vi "car.vi"() -> ()   [LabVIEW 2022 SP3]
uses:
  Control 1.ctl
  Control 2.ctl
  chicken.ctl
  plus_one.ctl
  game_over.ctl
  Control 4.ctl
  tree_control.ctl
panel:
  out "Boolean 12":T1
  in  "chicken":T2
  in  "tree 2":T3
  in  "tree":T3
  in  "tree 5":T3
  in  "tree 4":T3
  out "TOP":i16
  out "SCORE":i16
  in  "stop":bool
  in  "tree 3":T3
  out "Boolean 11":T4
  out "grass 5":T5
  out "grass 4":T5
  out "grass 3":T5
  out "grass 2":T5
  out "grass 1":T5
  out "easy?":bool
  in  "HARD":bool
  in  "EASY":bool
  out "Boolean 10":T6
  in  "v 10":dbl
  in  "v 9":dbl
  out "Boolean 9":T7
  in  "v 8":dbl
  out "Boolean 8":T6
  in  "v 7":dbl
  out "Boolean 7":T7
  out "Boolean 6":T6
  in  "v 6":dbl
  in  "v 5":dbl
  out "Boolean 5":T7
  in  "v 4":dbl
  out "Boolean 4":T6
  in  "v 3":dbl
  out "Boolean 3":T7
  in  "v 2":dbl
  in  "v":dbl
  out "Boolean 2":T6
  out "Boolean":T7
  # "SCORE"
  # "TOP"
  # "Press Arrow Key To Control The Chick\nDon't forget to reset the path of music first."
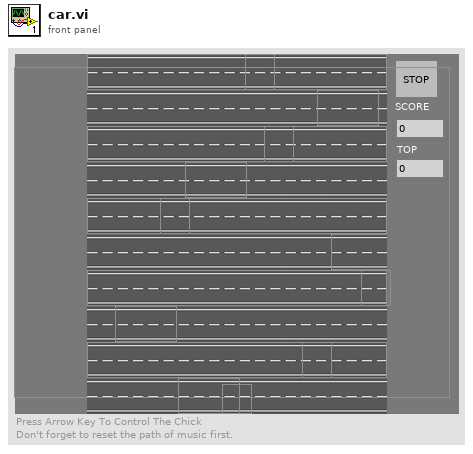
[diagram p1: front panel]
types:
  T1 = typedef "game_over.ctl" = bool
  T2 = typedef "chicken.ctl" = bool
  T3 = typedef "tree_control.ctl" = bool
  T4 = typedef "plus_one.ctl" = bool
  T5 = typedef "Control 4.ctl" = bool
  T6 = typedef "Control 2.ctl" = bool
  T7 = typedef "Control 1.ctl" = bool
  T8 = typedef "Sound Output Task ID.ctl" = u32
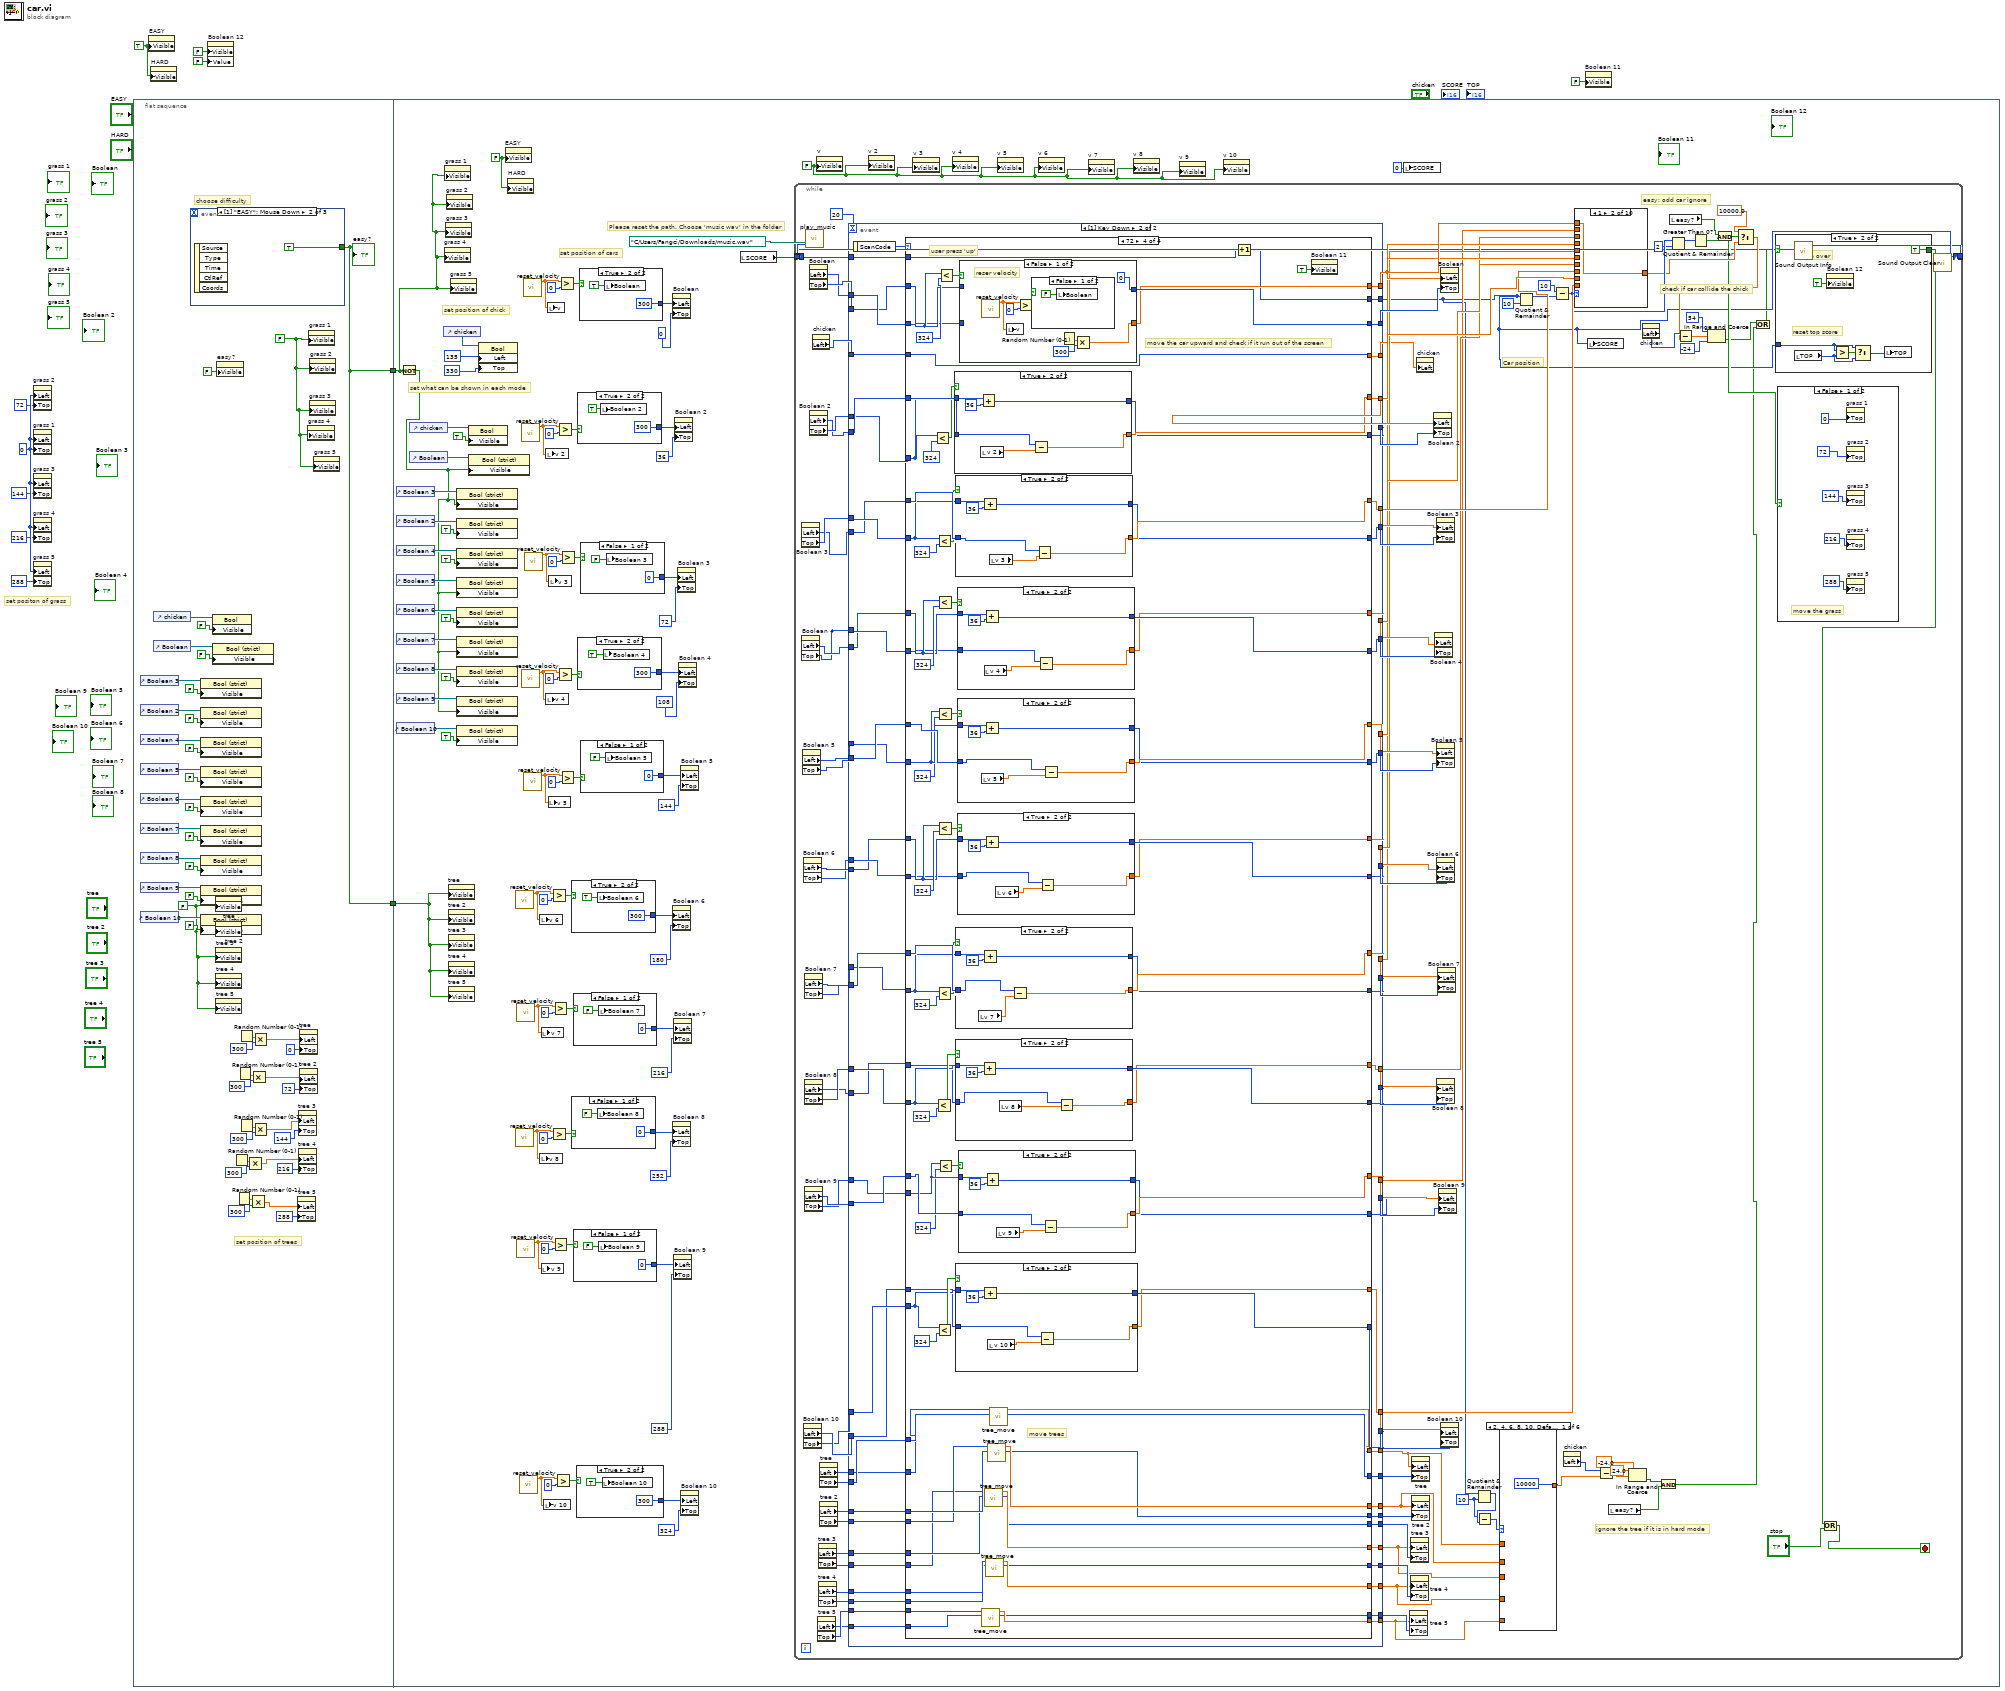
[diagram p0: block diagram]
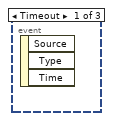
[diagram p2: hidden frame]
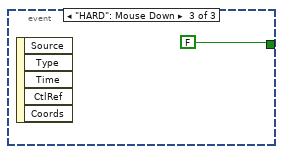
[diagram p3: hidden frame]
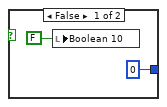
[diagram p4: hidden frame]
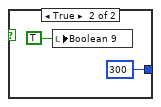
[diagram p5: hidden frame]
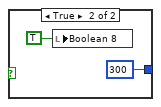
[diagram p6: hidden frame]
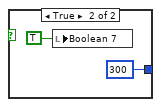
[diagram p7: hidden frame]
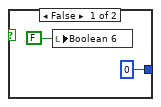
[diagram p8: hidden frame]
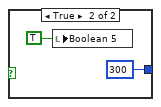
[diagram p9: hidden frame]
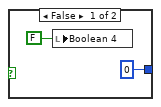
[diagram p10: hidden frame]
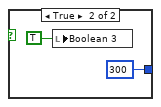
[diagram p11: hidden frame]
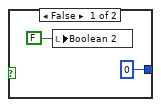
[diagram p12: hidden frame]
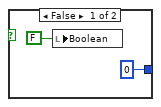
[diagram p13: hidden frame]
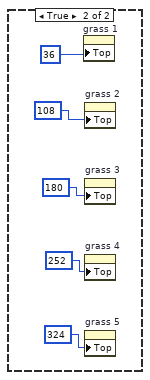
[diagram p19: hidden frame]
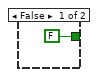
[diagram p20: hidden frame]
diagram:
  w6 = 0
  w8 = TRUE ("Visible")
  # "set positon of grass"
  n1 = property on="grass 2" class="Bool"("Left"=w6, "Top"=72) -> ()  [unwired: 2 in, 2 out]
  n2 = property on="grass 1" class="Bool"("Left"=w6, "Top"=w6) -> ()  [unwired: 2 in, 2 out]
  n3 = property on="grass 3" class="Bool"("Left"=w6, "Top"=144) -> ()  [unwired: 2 in, 2 out]
  n4 = property on="grass 4" class="Bool"("Left"=w6, "Top"=216) -> ()  [unwired: 2 in, 2 out]
  n5 = property on="grass 5" class="Bool"("Left"=w6, "Top"=288) -> ()  [unwired: 2 in, 2 out]
  n6 = flat-sequence {
    tunnel: [w32] -> w7
    tunnel: [w32] -> w1
    tunnel: w7 -> [w65]
    tunnel: w1 -> [w63]
    frame #0 {
      w33 = FALSE
      w34 = FALSE ("Visible")
      # "set position of trees"
      # "choose difficulty"
      n7 = control-ref of="Boolean 3"() -> (w44:refnum<vi>)
      n8 = control-ref of="Boolean 2"() -> (w43:refnum<vi>)
      n9 = control-ref of="Boolean 4"() -> (w42:refnum<vi>)
      n10 = control-ref of="Boolean 5"() -> (w41:refnum<vi>)
      n11 = control-ref of="Boolean 6"() -> (w40:refnum<vi>)
      n12 = control-ref of="Boolean 7"() -> (w39:refnum<vi>)
      n13 = control-ref of="Boolean 8"() -> (w38:refnum<vi>)
      n14 = control-ref of="Boolean 9"() -> (w37:refnum<vi>)
      n15 = control-ref of="Boolean 10"() -> (w35:refnum<vi>)
      n16 = control-ref of="chicken"() -> (w56:refnum<vi>)
      n17 = control-ref of="Boolean"() -> (w45:refnum<vi>)
      n18 = event shown="[1] \"EASY\": Mouse Down" {
        selector: _ -> [_ _ _]
        dyn-events: _ -> [_ _ _]
        timeout: _ -> [_ _ _]
        tunnel: [_ TRUE FALSE] -> w32
        event Timeout {
          n19 = event-data() -> ()  [unwired: 1 in, 3 out]
        }
        event "EASY": Mouse Down {
          n20 = event-data() -> ()  [unwired: 1 in, 5 out]
        }
        event "HARD": Mouse Down {
          n21 = event-data() -> ()  [unwired: 1 in, 5 out]
        }
      }
      "easy?" <- w32
      n22 = property class="Bool (strict)"(reference=w44, "Visible"=FALSE) -> ()  [unwired: 1 in, 2 out]
      n23 = property class="Bool (strict)"(reference=w43, "Visible"=FALSE) -> ()  [unwired: 1 in, 2 out]
      n24 = property class="Bool (strict)"(reference=w42, "Visible"=FALSE) -> ()  [unwired: 1 in, 2 out]
      n25 = property class="Bool (strict)"(reference=w41, "Visible"=FALSE) -> ()  [unwired: 1 in, 2 out]
      n26 = property class="Bool (strict)"(reference=w40, "Visible"=FALSE) -> ()  [unwired: 1 in, 2 out]
      n27 = property class="Bool (strict)"(reference=w39, "Visible"=FALSE) -> ()  [unwired: 1 in, 2 out]
      n28 = property class="Bool (strict)"(reference=w38, "Visible"=FALSE) -> ()  [unwired: 1 in, 2 out]
      n29 = property class="Bool (strict)"(reference=w37, "Visible"=FALSE) -> ()  [unwired: 1 in, 2 out]
      n30 = property class="Bool (strict)"(reference=w35, "Visible"=FALSE) -> ()  [unwired: 1 in, 2 out]
      n31 = property class="Bool"(reference=w56, "Visible"=FALSE) -> ()  [unwired: 1 in, 2 out]
      n32 = property class="Bool (strict)"(reference=w45, "Visible"=FALSE) -> ()  [unwired: 1 in, 2 out]
      n33 = property on="tree" class="Bool"("Visible"=w33) -> ()  [unwired: 2 in, 2 out]
      n34 = property on="tree 2" class="Bool"("Visible"=w33) -> ()  [unwired: 2 in, 2 out]
      n35 = property on="tree 3" class="Bool"("Visible"=w33) -> ()  [unwired: 2 in, 2 out]
      n36 = property on="tree 4" class="Bool"("Visible"=w33) -> ()  [unwired: 2 in, 2 out]
      n37 = property on="tree 5" class="Bool"("Visible"=w33) -> ()  [unwired: 2 in, 2 out]
      n38 = property on="easy?" class="Bool (strict)"("Visible"=FALSE) -> ()  [unwired: 2 in, 2 out]
      n39 = Random Number (0-1)() -> (number: 0 to 1=w23:dbl)
      n40 = Random Number (0-1)() -> (number: 0 to 1=w22:dbl)
      n41 = Random Number (0-1)() -> (number: 0 to 1=w27:dbl)
      n42 = Random Number (0-1)() -> (number: 0 to 1=w31:dbl)
      n43 = Random Number (0-1)() -> (number: 0 to 1=w26:dbl)
      n44 = Multiply(x=w23, y=300) -> (x*y=w18:dbl)
      n45 = Multiply(x=w22, y=300) -> (x*y=w17:dbl)
      n46 = Multiply(x=w27, y=300) -> (x*y=w20:dbl)
      n47 = Multiply(x=w31, y=300) -> (x*y=w29:dbl)
      n48 = Multiply(x=w26, y=300) -> (x*y=w19:dbl)
      n49 = property on="tree 5" class="Bool"("Left"=w17, "Top"=288 ("Position:Top")) -> ()  [unwired: 2 in, 2 out]
      n50 = property on="tree 3" class="Bool"("Left"=w19, "Top"=144 ("Position:Top")) -> ()  [unwired: 2 in, 2 out]
      n51 = property on="tree 4" class="Bool"("Left"=w18, "Top"=216 ("Position:Top")) -> ()  [unwired: 2 in, 2 out]
      n52 = property on="tree" class="Bool"("Left"=w29, "Top"=0 ("Position:Top")) -> ()  [unwired: 2 in, 2 out]
      n53 = property on="tree 2" class="Bool"("Left"=w20, "Top"=72 ("Position:Top")) -> ()  [unwired: 2 in, 2 out]
      n54 = property on="grass 4" class="Bool"("Visible"=w34) -> ()  [unwired: 2 in, 2 out]
      n55 = property on="grass 1" class="Bool"("Visible"=w34) -> ()  [unwired: 2 in, 2 out]
      n56 = property on="grass 3" class="Bool"("Visible"=w34) -> ()  [unwired: 2 in, 2 out]
      n57 = property on="grass 2" class="Bool"("Visible"=w34) -> ()  [unwired: 2 in, 2 out]
      n58 = property on="grass 5" class="Bool"("Visible"=w34) -> ()  [unwired: 2 in, 2 out]
    }
    frame #1 {
      w84 = FALSE ("Visible")
      w98 = FALSE ("Visible")
      # "Please reset the path. Choose 'music wav' in the folder"
      # "set position of cars"
      # "set position of chick"
      # "set what can be shown in each mode"
      n59 = control-ref of="Boolean 3"() -> (w74:refnum<vi>)
      n60 = control-ref of="Boolean 2"() -> (w75:refnum<vi>)
      n61 = control-ref of="Boolean 4"() -> (w76:refnum<vi>)
      n62 = control-ref of="Boolean 5"() -> (w77:refnum<vi>)
      n63 = control-ref of="Boolean 6"() -> (w78:refnum<vi>)
      n64 = control-ref of="Boolean 7"() -> (w79:refnum<vi>)
      n65 = control-ref of="Boolean 8"() -> (w80:refnum<vi>)
      n66 = control-ref of="Boolean 9"() -> (w81:refnum<vi>)
      n67 = control-ref of="Boolean 10"() -> (w83:refnum<vi>)
      n68 = Not(x=w65) -> (.not. x?=w66:bool)
      n69 = control-ref of="chicken"() -> (w67:refnum<vi>)
      n70 = control-ref of="Boolean"() -> (w73:refnum<vi>)
      n71 = control-ref of="chicken"() -> (w88:refnum<vi>)
      n72 = property on="grass 4" class="Bool"("Visible"=w65) -> ()  [unwired: 2 in, 2 out]
      n73 = property on="grass 1" class="Bool"("Visible"=w65) -> ()  [unwired: 2 in, 2 out]
      n74 = property on="grass 3" class="Bool"("Visible"=w65) -> ()  [unwired: 2 in, 2 out]
      n75 = property on="grass 2" class="Bool"("Visible"=w65) -> ()  [unwired: 2 in, 2 out]
      n76 = property on="tree" class="Bool"("Visible"=w63) -> ()  [unwired: 2 in, 2 out]
      n77 = property on="tree 2" class="Bool"("Visible"=w63) -> ()  [unwired: 2 in, 2 out]
      n78 = property on="tree 3" class="Bool"("Visible"=w63) -> ()  [unwired: 2 in, 2 out]
      n79 = property on="tree 4" class="Bool"("Visible"=w63) -> ()  [unwired: 2 in, 2 out]
      n80 = property on="tree 5" class="Bool"("Visible"=w63) -> ()  [unwired: 2 in, 2 out]
      n81 = property on="grass 5" class="Bool"("Visible"=w65) -> ()  [unwired: 2 in, 2 out]
      n82 = property class="Bool (strict)"(reference=w74, "Visible"=w66) -> ()  [unwired: 1 in, 2 out]
      n83 = property class="Bool (strict)"(reference=w75, "Visible"=TRUE) -> ()  [unwired: 1 in, 2 out]
      n84 = property class="Bool (strict)"(reference=w76, "Visible"=TRUE) -> ()  [unwired: 1 in, 2 out]
      n85 = property class="Bool (strict)"(reference=w77, "Visible"=w66) -> ()  [unwired: 1 in, 2 out]
      n86 = property class="Bool (strict)"(reference=w78, "Visible"=TRUE) -> ()  [unwired: 1 in, 2 out]
      n87 = property class="Bool (strict)"(reference=w79, "Visible"=w66) -> ()  [unwired: 1 in, 2 out]
      n88 = property class="Bool (strict)"(reference=w80, "Visible"=TRUE) -> ()  [unwired: 1 in, 2 out]
      n89 = property class="Bool (strict)"(reference=w81, "Visible"=w66) -> ()  [unwired: 1 in, 2 out]
      n90 = property class="Bool (strict)"(reference=w83, "Visible"=TRUE) -> ()  [unwired: 1 in, 2 out]
      n91 = property class="Bool"(reference=w67, "Visible"=TRUE) -> ()  [unwired: 1 in, 2 out]
      n92 = property class="Bool (strict)"(reference=w73, "Visible"=w66) -> ()  [unwired: 1 in, 2 out]
      n93 = property on="Property Node" class="Bool"(reference=w88, "Left"=135 ("Position:Left"), "Top"=330 ("Position:Top")) -> ()  [unwired: 1 in, 2 out]
      n94 = property on="EASY" class="Bool"("Visible"=w84) -> ()  [unwired: 2 in, 2 out]
      n95 = property on="HARD" class="Bool"("Visible"=w84) -> ()  [unwired: 2 in, 2 out]
      n96 = call "reset_velocity.vi"() -> ("Numeric"=w93:dbl)  [unwired: 11 in]
      n97 = call "reset_velocity.vi"() -> ("Numeric"=w91:dbl)  [unwired: 11 in]
      n98 = call "reset_velocity.vi"() -> ("Numeric"=w92:dbl)  [unwired: 11 in]
      n99 = call "reset_velocity.vi"() -> ("Numeric"=w90:dbl)  [unwired: 11 in]
      n100 = call "reset_velocity.vi"() -> ("Numeric"=w89:dbl)  [unwired: 11 in]
      n101 = call "reset_velocity.vi"() -> ("Numeric"=w97:dbl)  [unwired: 11 in]
      n102 = call "reset_velocity.vi"() -> ("Numeric"=w95:dbl)  [unwired: 11 in]
      n103 = call "reset_velocity.vi"() -> ("Numeric"=w139:dbl)  [unwired: 11 in]
      n104 = call "reset_velocity.vi"() -> ("Numeric"=w94:dbl)  [unwired: 11 in]
      n105 = call "reset_velocity.vi"() -> ("Numeric"=w96:dbl)  [unwired: 11 in]
      n106 = local write "v 6"(w93) -> ()
      n107 = local write "v 8"(w91) -> ()
      n108 = local write "v 7"(w92) -> ()
      n109 = local write "v 9"(w90) -> ()
      n110 = local write "v 10"(w89) -> ()
      n111 = local write "v 2"(w97) -> ()
      n112 = local write "v 4"(w95) -> ()
      n113 = local write "v"(w139) -> ()
      n114 = local write "v 5"(w94) -> ()
      n115 = local write "v 3"(w96) -> ()
      n116 = Greater?(x=w93, y=0) -> (0:w118:bool)
      n117 = Greater?(x=w91, y=0) -> (0:w110:bool)
      n118 = Greater?(x=w92, y=0) -> (0:w113:bool)
      n119 = Greater?(x=w90, y=0) -> (0:w105:bool)
      n120 = Greater?(x=w89, y=0) -> (0:w102:bool)
      n121 = Greater?(x=w97, y=0) -> (0:w134:bool)
      n122 = Greater?(x=w95, y=0) -> (0:w126:bool)
      n123 = Greater?(x=w139, y=0) -> (0:w137:bool)
      n124 = Greater?(x=w94, y=0) -> (0:w121:bool)
      n125 = Greater?(x=w96, y=0) -> (0:w129:bool)
      n126 = case shown="True" w118 {
        tunnel: [0 300] -> w116
        frame False {
          n127 = local write "Boolean 6"(FALSE) -> ()
        }
        frame True {
          n128 = local write "Boolean 6"(TRUE) -> ()
        }
      }
      n129 = case shown="False" w110 {
        tunnel: [0 300] -> w108
        frame False {
          n130 = local write "Boolean 8"(FALSE) -> ()
        }
        frame True {
          n131 = local write "Boolean 8"(TRUE) -> ()
        }
      }
      n132 = case shown="False" w113 {
        tunnel: [0 300] -> w112
        frame False {
          n133 = local write "Boolean 7"(FALSE) -> ()
        }
        frame True {
          n134 = local write "Boolean 7"(TRUE) -> ()
        }
      }
      n135 = case shown="False" w105 {
        tunnel: [0 300] -> w104
        frame False {
          n136 = local write "Boolean 9"(FALSE) -> ()
        }
        frame True {
          n137 = local write "Boolean 9"(TRUE) -> ()
        }
      }
      n138 = case shown="True" w102 {
        tunnel: [0 300] -> w100
        frame False {
          n139 = local write "Boolean 10"(FALSE) -> ()
        }
        frame True {
          n140 = local write "Boolean 10"(TRUE) -> ()
        }
      }
      n141 = case shown="True" w134 {
        tunnel: [0 300] -> w132
        frame False {
          n142 = local write "Boolean 2"(FALSE) -> ()
        }
        frame True {
          n143 = local write "Boolean 2"(TRUE) -> ()
        }
      }
      n144 = case shown="True" w126 {
        tunnel: [0 300] -> w124
        frame False {
          n145 = local write "Boolean 4"(FALSE) -> ()
        }
        frame True {
          n146 = local write "Boolean 4"(TRUE) -> ()
        }
      }
      n147 = case shown="True" w137 {
        tunnel: [0 300] -> w136
        frame False {
          n148 = local write "Boolean"(FALSE) -> ()
        }
        frame True {
          n149 = local write "Boolean"(TRUE) -> ()
        }
      }
      n150 = case shown="False" w121 {
        tunnel: [0 300] -> w120
        frame False {
          n151 = local write "Boolean 5"(FALSE) -> ()
        }
        frame True {
          n152 = local write "Boolean 5"(TRUE) -> ()
        }
      }
      n153 = case shown="False" w129 {
        tunnel: [0 300] -> w127
        frame False {
          n154 = local write "Boolean 3"(FALSE) -> ()
        }
        frame True {
          n155 = local write "Boolean 3"(TRUE) -> ()
        }
      }
      n156 = property on="Boolean" class="Bool (strict)"("Left"=w136, "Top"=0) -> ()  [unwired: 2 in, 2 out]
      n157 = property on="Boolean 6" class="Bool (strict)"("Left"=w116, "Top"=180) -> ()  [unwired: 2 in, 2 out]
      n158 = property on="Boolean 8" class="Bool (strict)"("Left"=w108, "Top"=252) -> ()  [unwired: 2 in, 2 out]
      n159 = property on="Boolean 7" class="Bool (strict)"("Left"=w112, "Top"=216) -> ()  [unwired: 2 in, 2 out]
      n160 = property on="Boolean 9" class="Bool (strict)"("Left"=w104, "Top"=288) -> ()  [unwired: 2 in, 2 out]
      n161 = property on="Boolean 2" class="Bool (strict)"("Left"=w132, "Top"=36) -> ()  [unwired: 2 in, 2 out]
      n162 = property on="Boolean 3" class="Bool (strict)"("Left"=w127, "Top"=72) -> ()  [unwired: 2 in, 2 out]
      n163 = property on="Boolean 4" class="Bool (strict)"("Left"=w124, "Top"=108) -> ()  [unwired: 2 in, 2 out]
      n164 = property on="Boolean 5" class="Bool (strict)"("Left"=w120, "Top"=144) -> ()  [unwired: 2 in, 2 out]
      n165 = property on="Boolean 10" class="Bool (strict)"("Left"=w100, "Top"=324) -> ()  [unwired: 2 in, 2 out]
      n166 = local read "SCORE"() -> (w64:i16)
      n167 = call "play_music.vi"("Sound File Path"=path "C:/Users/Fangci/Downloads/music.wav") -> ("task ID"=w61:T8)  [unwired: 10 in]
      n168 = while {
        shift-right: [w201] -> _
        shift-left: w64 -> [w217]
        tunnel: w61 -> [w181]
        tunnel: [w180] -> w60
        stop <- w182 stop-if-true
        w199 = i16 10 ("y")
        # "ignore the tree if it is in hard mode"
        # "check if car collide the chick"
        # "easy: odd car ignore"
        # "Car position"
        n169 = property on="Boolean 3" class="Bool (strict)"() -> ("Left"=w270:i32, "Top"=w271:i32)  [unwired: 2 in, 2 out]
        n170 = property on="Boolean 4" class="Bool (strict)"() -> ("Left"=w268:i32, "Top"=w267:i32)  [unwired: 2 in, 2 out]
        n171 = property on="Boolean 5" class="Bool (strict)"() -> ("Left"=w257:i32, "Top"=w265:i32)  [unwired: 2 in, 2 out]
        n172 = property on="Boolean 6" class="Bool (strict)"() -> ("Left"=w263:i32, "Top"=w262:i32)  [unwired: 2 in, 2 out]
        n173 = property on="Boolean 10" class="Bool (strict)"() -> ("Left"=w250:i32, "Top"=w249:i32)  [unwired: 2 in, 2 out]
        n174 = property on="Boolean 7" class="Bool (strict)"() -> ("Left"=w256:i32, "Top"=w260:i32)  [unwired: 2 in, 2 out]
        n175 = property on="Boolean 8" class="Bool (strict)"() -> ("Left"=w255:i32, "Top"=w258:i32)  [unwired: 2 in, 2 out]
        n176 = property on="Boolean 9" class="Bool (strict)"() -> ("Left"=w253:i32, "Top"=w252:i32)  [unwired: 2 in, 2 out]
        n177 = property on="Boolean" class="Bool (strict)"() -> ("Left"=w276:i32, "Top"=w277:i32)  [unwired: 2 in, 2 out]
        n178 = property on="Boolean 2" class="Bool (strict)"() -> ("Left"=w274:i32, "Top"=w275:i32)  [unwired: 2 in, 2 out]
        n179 = property on="chicken" class="Bool"() -> ("Left"=w221:i32)  [unwired: 2 in, 2 out]
        n180 = property on="tree 5" class="Bool"() -> ("Left"=w206:i32, "Top"=w207:i32)  [unwired: 2 in, 2 out]
        n181 = property on="tree 3" class="Bool"() -> ("Left"=w211:i32, "Top"=w210:i32)  [unwired: 2 in, 2 out]
        n182 = property on="tree 4" class="Bool"() -> ("Left"=w208:i32, "Top"=w209:i32)  [unwired: 2 in, 2 out]
        n183 = property on="tree" class="Bool"() -> ("Left"=w215:i32, "Top"=w216:i32)  [unwired: 2 in, 2 out]
        n184 = property on="tree 2" class="Bool"() -> ("Left"=w213:i32, "Top"=w212:i32)  [unwired: 2 in, 2 out]
        n185 = event shown="[1] Key Down" {
          selector: _ -> [_ _]
          dyn-events: _ -> [_ _]
          timeout: 20 -> [_ _]
          tunnel: [w397 w558] -> w272
          tunnel: [w399 w556] -> w246
          tunnel: w276 -> [w398 w555]
          tunnel: w277 -> [w397 w557]
          tunnel: [w396 w551] -> w273
          tunnel: [w394 w552] -> w245
          tunnel: w274 -> [w395 w554]
          tunnel: w275 -> [w396 w553]
          tunnel: [w388 w547] -> w269
          tunnel: [w386 w548] -> w244
          tunnel: w270 -> [w387 w549]
          tunnel: w271 -> [w388 w550]
          tunnel: [w373 w543] -> w266
          tunnel: [w375 w544] -> w243
          tunnel: w268 -> [w374 w545]
          tunnel: w267 -> [w373 w546]
          tunnel: [w372 w540] -> w264
          tunnel: [w370 w539] -> w242
          tunnel: w257 -> [w371 w542]
          tunnel: w265 -> [w372 w541]
          tunnel: [w357 w535] -> w261
          tunnel: [w359 w536] -> w241
          tunnel: w263 -> [w358 w537]
          tunnel: w262 -> [w357 w538]
          tunnel: [w356 w531] -> w259
          tunnel: [w354 w532] -> w240
          tunnel: w256 -> [w355 w534]
          tunnel: w260 -> [w356 w533]
          tunnel: [w341 w527] -> w254
          tunnel: [w343 w528] -> w239
          tunnel: w255 -> [w342 w529]
          tunnel: w258 -> [w341 w530]
          tunnel: [w340 w523] -> w251
          tunnel: [w338 w524] -> w238
          tunnel: w253 -> [w339 w526]
          tunnel: w252 -> [w340 w525]
          tunnel: [w325 w519] -> w248
          tunnel: [w327 w520] -> w237
          tunnel: w250 -> [w326 w521]
          tunnel: w249 -> [w325 w522]
          tunnel: w221 -> [w323 w518]
          tunnel: [w323 w517] -> w220
          tunnel: w217 -> [w322 w516]
          tunnel: [w322 w515] -> w201
          tunnel: w216 -> [w320 w514]
          tunnel: w215 -> [w321 w513]
          tunnel: [w320 w512] -> w214
          tunnel: [w321 w511] -> w197
          tunnel: w213 -> [w319 w510]
          tunnel: w212 -> [w318 w509]
          tunnel: w211 -> [w317 w508]
          tunnel: w210 -> [w316 w507]
          tunnel: w209 -> [w314 w506]
          tunnel: w208 -> [w315 w505]
          tunnel: w207 -> [w313 w504]
          tunnel: w206 -> [w312 w503]
          tunnel: [w319 w502] -> w196
          tunnel: [w318 w501] -> w205
          tunnel: [w317 w500] -> w195
          tunnel: [w316 w499] -> w204
          tunnel: [w315 w498] -> w194
          tunnel: [w314 w497] -> w203
          tunnel: [w312 w496] -> w193
          tunnel: [w313 w495] -> w202
          event Timeout {
            # "if the car run over the range of screen, reser the velocity"
            # "move cars"
            n186 = event-data() -> ()  [unwired: 1 in, 1 out]
            n187 = Greater Or Equal?(x=w398, y=-62) -> (x >= y?=w403:bool)
            n188 = Less Or Equal?(x=w398, y=300) -> (x <= y?=w404:bool)
            n189 = Greater Or Equal?(x=w395, y=-62) -> (x >= y?=w390:bool)
            n190 = Greater Or Equal?(x=w371, y=-62) -> (x >= y?=w366:bool)
            n191 = Less Or Equal?(x=w395, y=300) -> (x <= y?=w389:bool)
            n192 = Greater Or Equal?(x=w387, y=-62) -> (x >= y?=w382:bool)
            n193 = Greater Or Equal?(x=w374, y=-62) -> (x >= y?=w379:bool)
            n194 = Less Or Equal?(x=w371, y=300) -> (x <= y?=w365:bool)
            n195 = Less Or Equal?(x=w387, y=300) -> (x <= y?=w381:bool)
            n196 = Less Or Equal?(x=w374, y=300) -> (x <= y?=w380:bool)
            n197 = Greater Or Equal?(x=w358, y=-62) -> (x >= y?=w363:bool)
            n198 = Less Or Equal?(x=w358, y=300) -> (x <= y?=w364:bool)
            n199 = Greater Or Equal?(x=w355, y=-62) -> (x >= y?=w350:bool)
            n200 = Greater Or Equal?(x=w342, y=-62) -> (x >= y?=w347:bool)
            n201 = Less Or Equal?(x=w355, y=300) -> (x <= y?=w349:bool)
            n202 = Less Or Equal?(x=w342, y=300) -> (x <= y?=w348:bool)
            n203 = Greater Or Equal?(x=w339, y=-62) -> (x >= y?=w334:bool)
            n204 = Less Or Equal?(x=w339, y=300) -> (x <= y?=w333:bool)
            n205 = Greater Or Equal?(x=w326, y=-62) -> (x >= y?=w331:bool)
            n206 = Less Or Equal?(x=w326, y=300) -> (x <= y?=w332:bool)
            n207 = And(x=w403, y=w404) -> (x .and. y?=w402:bool)
            n208 = And(x=w390, y=w389) -> (x .and. y?=w391:bool)
            n209 = And(x=w366, y=w365) -> (x .and. y?=w367:bool)
            n210 = And(x=w382, y=w381) -> (x .and. y?=w383:bool)
            n211 = And(x=w379, y=w380) -> (x .and. y?=w378:bool)
            n212 = And(x=w363, y=w364) -> (x .and. y?=w362:bool)
            n213 = And(x=w350, y=w349) -> (x .and. y?=w351:bool)
            n214 = And(x=w347, y=w348) -> (x .and. y?=w346:bool)
            n215 = And(x=w334, y=w333) -> (x .and. y?=w335:bool)
            n216 = And(x=w331, y=w332) -> (x .and. y?=w330:bool)
            n217 = case shown="True" w402 {
              tunnel: [w486 w493] -> w399
              tunnel: w398 -> [_ w492]
              frame False {
                n218 = local read "v"() -> (w489:dbl)
                n219 = Greater?(x=w489, y=0) -> (0:w487:bool)
                n220 = case shown="False" w487 {
                  tunnel: [0 300] -> w486
                  frame False {
                  }
                  frame True {
                  }
                }
              }
              frame True {
                n221 = Subtract(x=w492, y="v") -> (x-y=w493:dbl)
              }
            }
            n222 = case shown="True" w391 {
              tunnel: [w477 w484] -> w394
              tunnel: w395 -> [_ w483]
              frame False {
                n223 = local read "v 2"() -> (w480:dbl)
                n224 = Greater?(x=w480, y=0) -> (0:w478:bool)
                n225 = case shown="False" w478 {
                  tunnel: [0 300] -> w477
                  frame False {
                  }
                  frame True {
                  }
                }
              }
              frame True {
                n226 = Subtract(x=w483, y="v 2") -> (x-y=w484:dbl)
              }
            }
            n227 = case shown="True" w367 {
              tunnel: [w450 w457] -> w370
              tunnel: w371 -> [_ w456]
              frame False {
                n228 = local read "v 5"() -> (w453:dbl)
                n229 = Greater?(x=w453, y=0) -> (0:w451:bool)
                n230 = case shown="False" w451 {
                  tunnel: [0 300] -> w450
                  frame False {
                  }
                  frame True {
                  }
                }
              }
              frame True {
                n231 = Subtract(x=w456, y="v 5") -> (x-y=w457:dbl)
              }
            }
            n232 = case shown="True" w383 {
              tunnel: [w468 w475] -> w386
              tunnel: w387 -> [_ w474]
              frame False {
                n233 = local read "v 3"() -> (w471:dbl)
                n234 = Greater?(x=w471, y=0) -> (0:w469:bool)
                n235 = case shown="False" w469 {
                  tunnel: [0 300] -> w468
                  frame False {
                  }
                  frame True {
                  }
                }
              }
              frame True {
                n236 = Subtract(x=w474, y="v 3") -> (x-y=w475:dbl)
              }
            }
            n237 = case shown="True" w378 {
              tunnel: [w459 w466] -> w375
              tunnel: w374 -> [_ w465]
              frame False {
                n238 = local read "v 4"() -> (w462:dbl)
                n239 = Greater?(x=w462, y=0) -> (0:w460:bool)
                n240 = case shown="False" w460 {
                  tunnel: [0 300] -> w459
                  frame False {
                  }
                  frame True {
                  }
                }
              }
              frame True {
                n241 = Subtract(x=w465, y="v 4") -> (x-y=w466:dbl)
              }
            }
            n242 = case shown="True" w362 {
              tunnel: [w441 w448] -> w359
              tunnel: w358 -> [_ w447]
              frame False {
                n243 = local read "v 6"() -> (w444:dbl)
                n244 = Greater?(x=w444, y=0) -> (0:w442:bool)
                n245 = case shown="False" w442 {
                  tunnel: [0 300] -> w441
                  frame False {
                  }
                  frame True {
                  }
                }
              }
              frame True {
                n246 = Subtract(x=w447, y="v 6") -> (x-y=w448:dbl)
              }
            }
            n247 = case shown="True" w351 {
              tunnel: [w432 w439] -> w354
              tunnel: w355 -> [_ w438]
              frame False {
                n248 = local read "v 7"() -> (w435:dbl)
                n249 = Greater?(x=w435, y=0) -> (0:w433:bool)
                n250 = case shown="False" w433 {
                  tunnel: [0 300] -> w432
                  frame False {
                  }
                  frame True {
                  }
                }
              }
              frame True {
                n251 = Subtract(x=w438, y="v 7") -> (x-y=w439:dbl)
              }
            }
            n252 = case shown="True" w346 {
              tunnel: [w423 w430] -> w343
              tunnel: w342 -> [_ w429]
              frame False {
                n253 = local read "v 8"() -> (w426:dbl)
                n254 = Greater?(x=w426, y=0) -> (0:w424:bool)
                n255 = case shown="False" w424 {
                  tunnel: [0 300] -> w423
                  frame False {
                  }
                  frame True {
                  }
                }
              }
              frame True {
                n256 = Subtract(x=w429, y="v 8") -> (x-y=w430:dbl)
              }
            }
            n257 = case shown="True" w335 {
              tunnel: [w414 w421] -> w338
              tunnel: w339 -> [_ w420]
              frame False {
                n258 = local read "v 9"() -> (w417:dbl)
                n259 = Greater?(x=w417, y=0) -> (0:w415:bool)
                n260 = case shown="False" w415 {
                  tunnel: [0 300] -> w414
                  frame False {
                  }
                  frame True {
                  }
                }
              }
              frame True {
                n261 = Subtract(x=w420, y="v 9") -> (x-y=w421:dbl)
              }
            }
            n262 = case shown="True" w330 {
              tunnel: [w405 w412] -> w327
              tunnel: w326 -> [_ w411]
              frame False {
                n263 = local read "v 10"() -> (w408:dbl)
                n264 = Greater?(x=w408, y=0) -> (0:w406:bool)
                n265 = case shown="False" w406 {
                  tunnel: [0 300] -> w405
                  frame False {
                  }
                  frame True {
                  }
                }
              }
              frame True {
                n266 = Subtract(x=w411, y="v 10") -> (x-y=w412:dbl)
              }
            }
            n267 = property on="Boolean 11" class="Bool (strict)"("Visible"=FALSE) -> ()  [unwired: 2 in, 2 out]
          }
          event Key Down {
            n268 = event-data() -> ("ScanCode"=w559:i16)  [unwired: 1 in]
            n269 = case shown="72" w559 {
              tunnel: [w591 w621 w658 w748] -> w558
              tunnel: w557 -> [w591 w621 w658 w747]
              tunnel: [w590 w622 w659 w746] -> w556
              tunnel: w555 -> [w590 w622 w659 w745]
              tunnel: [w588 w603 w656 w741] -> w551
              tunnel: w553 -> [w588 w603 w656 w742]
              tunnel: [w589 w604 w657 w743] -> w552
              tunnel: w554 -> [w589 w604 w657 w744]
              tunnel: [w586 w620 w654 w735] -> w547
              tunnel: w550 -> [w586 w620 w654 w736]
              tunnel: [w587 w619 w655 w737] -> w548
              tunnel: w549 -> [w587 w619 w655 w738]
              tunnel: [w584 w617 w652 w730] -> w543
              tunnel: w546 -> [w584 w617 w652 w729]
              tunnel: [w585 w618 w653 w728] -> w544
              tunnel: w545 -> [w585 w618 w653 w727]
              tunnel: [w582 w615 w650 w723] -> w540
              tunnel: w541 -> [w582 w615 w650 w724]
              tunnel: [w583 w616 w651 w725] -> w539
              tunnel: w542 -> [w583 w616 w651 w726]
              tunnel: [w580 w613 w648 w718] -> w535
              tunnel: w538 -> [w580 w613 w648 w717]
              tunnel: [w581 w614 w649 w716] -> w536
              tunnel: w537 -> [w581 w614 w649 w715]
              tunnel: [w578 w611 w646 w711] -> w531
              tunnel: w533 -> [w578 w611 w646 w712]
              tunnel: [w579 w612 w647 w713] -> w532
              tunnel: w534 -> [w579 w612 w647 w714]
              tunnel: [w576 w609 w644 w706] -> w527
              tunnel: w530 -> [w576 w609 w644 w705]
              tunnel: [w577 w610 w645 w704] -> w528
              tunnel: w529 -> [w577 w610 w645 w703]
              tunnel: [w574 w607 w642 w699] -> w523
              tunnel: w525 -> [w574 w607 w642 w700]
              tunnel: [w575 w608 w643 w701] -> w524
              tunnel: w526 -> [w575 w608 w643 w702]
              tunnel: [w572 w605 w640 w694] -> w519
              tunnel: w522 -> [w572 w605 w640 w693]
              tunnel: [w573 w606 w641 w692] -> w520
              tunnel: w521 -> [w573 w606 w641 w691]
              tunnel: w518 -> [w571 w628 w663 w689]
              tunnel: [w571 w623 w660 w689] -> w517
              tunnel: w516 -> [w570 w602 w639 w688]
              tunnel: [w570 w602 w639 w687] -> w515
              tunnel: w514 -> [w569 w601 w638 w686]
              tunnel: w513 -> [w568 w600 w631 w685]
              tunnel: [w569 w601 w638 w684] -> w512
              tunnel: [w568 w600 w631 w683] -> w511
              tunnel: w510 -> [w567 w599 w637 w682]
              tunnel: w509 -> [w566 w598 w636 w681]
              tunnel: w508 -> [w565 w597 w635 w680]
              tunnel: w507 -> [w564 w596 w634 w679]
              tunnel: w506 -> [w562 w594 w632 w678]
              tunnel: w505 -> [w563 w595 w633 w677]
              tunnel: w504 -> [w561 w593 w629 w676]
              tunnel: w503 -> [w560 w592 w630 w675]
              tunnel: [w567 w599 w637 w674] -> w502
              tunnel: [w566 w598 w636 w673] -> w501
              tunnel: [w565 w597 w635 w672] -> w500
              tunnel: [w564 w596 w634 w671] -> w499
              tunnel: [w563 w595 w633 w670] -> w498
              tunnel: [w562 w594 w632 w669] -> w497
              tunnel: [w560 w592 w630 w668] -> w496
              tunnel: [w561 w593 w629 w667] -> w495
              frame 0, Default {
              }
              frame 75 {
                # "move chick"
                # "user press 'left'"
                n270 = Subtract(x=w628, y=20) -> (x-y=w624:i32)
                n271 = Less Than 0?(x=w624) -> (x < 0?=w626:bool)
                n272 = Select(t=0.0, s=w626, f=w624) -> (s? t:f=w623:dbl)
              }
              frame 77 {
                # "move chick"
                # "user press 'right'"
                n273 = Add(x=w663, y=20) -> (x+y=w662:i32)
                n274 = Greater?(x=w662, y=270) -> (0:w665:bool)
                n275 = Select(t=270.0, s=w665, f=w662) -> (s? t:f=w660:dbl)
              }
              frame 72 {
                # "move trees"
                # "move the car upward and check if it run out of the screen"
                # "user press 'up'"
                n276 = Less?(x=w742, y=324) -> (x < y?=w739:bool)
                n277 = Less?(x=w705, y=324) -> (x < y?=w708:bool)
                n278 = Less?(x=w736, y=324) -> (x < y?=w733:bool)
                n279 = Less?(x=w712, y=324) -> (x < y?=w709:bool)
                n280 = Less?(x=w693, y=324) -> (x < y?=w696:bool)
                n281 = Less?(x=w729, y=324) -> (x < y?=w732:bool)
                n282 = Less?(x=w724, y=324) -> (x < y?=w721:bool)
                n283 = Less?(x=w717, y=324) -> (x < y?=w720:bool)
                n284 = Less?(x=w700, y=324) -> (x < y?=w697:bool)
                n285 = Less?(x=w747, y=324) -> (x < y?=w750:bool)
                n286 = case shown="True" w739 {
                  tunnel: [0 w885] -> w741
                  tunnel: w742 -> [_ w884]
                  tunnel: [w871 w882] -> w743
                  tunnel: w744 -> [_ w881]
                  frame False {
                    n287 = call "reset_velocity.vi"() -> ("Numeric"=w874:dbl)  [unwired: 11 in]
                    n288 = local write "v 2"(w874) -> ()
                    n289 = Greater?(x=w874, y=0) -> (0:w876:bool)
                    n290 = case shown="False" w876 {
                      frame False {
                        n291 = local write "Boolean 2"(FALSE) -> ()
                      }
                      frame True {
                        n292 = local write "Boolean 2"(TRUE) -> ()
                      }
                    }
                    n293 = Random Number (0-1)() -> (number: 0 to 1=w873:dbl)
                    n294 = Multiply(x=w873, y=300) -> (x*y=w871:dbl)
                  }
                  frame True {
                    n295 = Add(x=w884, y=36) -> (x+y=w885:i32)
                    n296 = local read "v 2"() -> (w880:dbl)
                    n297 = Subtract(x=w881, y=w880) -> (x-y=w882:dbl)
                  }
                }
                n298 = case shown="True" w708 {
                  tunnel: [0 w795] -> w706
                  tunnel: w705 -> [_ w794]
                  tunnel: [w781 w791] -> w704
                  tunnel: w703 -> [_ w792]
                  frame False {
                    n299 = call "reset_velocity.vi"() -> ("Numeric"=w784:dbl)  [unwired: 11 in]
                    n300 = local write "v 8"(w784) -> ()
                    n301 = Greater?(x=w784, y=0) -> (0:w786:bool)
                    n302 = case shown="False" w786 {
                      frame False {
                        n303 = local write "Boolean 8"(FALSE) -> ()
                      }
                      frame True {
                        (unwired) 300
                        n304 = local write "Boolean 8"(TRUE) -> ()
                      }
                    }
                    n305 = Random Number (0-1)() -> (number: 0 to 1=w782:dbl)
                    n306 = Multiply(x=w782, y=300) -> (x*y=w781:dbl)
                  }
                  frame True {
                    n307 = Add(x=w794, y=36) -> (x+y=w795:i32)
                    n308 = local read "v 8"() -> (w790:dbl)
                    n309 = Subtract(x=w792, y=w790) -> (x-y=w791:dbl)
                  }
                }
                n310 = case shown="True" w733 {
                  tunnel: [0 w870] -> w735
                  tunnel: w736 -> [_ w869]
                  tunnel: [w856 w866] -> w737
                  tunnel: w738 -> [_ w867]
                  frame False {
                    n311 = call "reset_velocity.vi"() -> ("Numeric"=w859:dbl)  [unwired: 11 in]
                    n312 = local write "v 3"(w859) -> ()
                    n313 = Greater?(x=w859, y=0) -> (0:w861:bool)
                    n314 = case shown="True" w861 {
                      frame False {
                        (unwired) 0
                        n315 = local write "Boolean 3"(FALSE) -> ()
                      }
                      frame True {
                        n316 = local write "Boolean 3"(TRUE) -> ()
                      }
                    }
                    n317 = Random Number (0-1)() -> (number: 0 to 1=w858:dbl)
                    n318 = Multiply(x=w858, y=300) -> (x*y=w856:dbl)
                  }
                  frame True {
                    n319 = Add(x=w869, y=36) -> (x+y=w870:i32)
                    n320 = local read "v 3"() -> (w865:dbl)
                    n321 = Subtract(x=w867, y=w865) -> (x-y=w866:dbl)
                  }
                }
                n322 = case shown="True" w709 {
                  tunnel: [0 w810] -> w711
                  tunnel: w712 -> [_ w809]
                  tunnel: [w796 w806] -> w713
                  tunnel: w714 -> [_ w807]
                  frame False {
                    n323 = call "reset_velocity.vi"() -> ("Numeric"=w799:dbl)  [unwired: 11 in]
                    n324 = local write "v 7"(w799) -> ()
                    n325 = Greater?(x=w799, y=0) -> (0:w801:bool)
                    n326 = case shown="True" w801 {
                      frame False {
                        (unwired) 0
                        n327 = local write "Boolean 7"(FALSE) -> ()
                      }
                      frame True {
                        n328 = local write "Boolean 7"(TRUE) -> ()
                      }
                    }
                    n329 = Random Number (0-1)() -> (number: 0 to 1=w798:dbl)
                    n330 = Multiply(x=w798, y=300) -> (x*y=w796:dbl)
                  }
                  frame True {
                    n331 = local read "v 7"() -> (w805:dbl)
                    n332 = Add(x=w809, y=36) -> (x+y=w810:i32)
                    n333 = Subtract(x=w807, y=w805) -> (x-y=w806:dbl)
                  }
                }
                n334 = case shown="True" w696 {
                  tunnel: [0 w765] -> w694
                  tunnel: w693 -> [_ w764]
                  tunnel: [w751 w761] -> w692
                  tunnel: w691 -> [_ w762]
                  frame False {
                    n335 = call "reset_velocity.vi"() -> ("Numeric"=w754:dbl)  [unwired: 11 in]
                    n336 = local write "v 10"(w754) -> ()
                    n337 = Greater?(x=w754, y=0) -> (0:w756:bool)
                    n338 = case shown="False" w756 {
                      frame False {
                        n339 = local write "Boolean 10"(FALSE) -> ()
                      }
                      frame True {
                        (unwired) 300
                        n340 = local write "Boolean 10"(TRUE) -> ()
                      }
                    }
                    n341 = Random Number (0-1)() -> (number: 0 to 1=w752:dbl)
                    n342 = Multiply(x=w752, y=300) -> (x*y=w751:dbl)
                  }
                  frame True {
                    n343 = Add(x=w764, y=36) -> (x+y=w765:i32)
                    n344 = local read "v 10"() -> (w760:dbl)
                    n345 = Subtract(x=w762, y=w760) -> (x-y=w761:dbl)
                  }
                }
                n346 = case shown="True" w732 {
                  tunnel: [0 w855] -> w730
                  tunnel: w729 -> [_ w854]
                  tunnel: [w841 w851] -> w728
                  tunnel: w727 -> [_ w852]
                  frame False {
                    n347 = call "reset_velocity.vi"() -> ("Numeric"=w844:dbl)  [unwired: 11 in]
                    n348 = local write "v 4"(w844) -> ()
                    n349 = Greater?(x=w844, y=0) -> (0:w846:bool)
                    n350 = case shown="False" w846 {
                      frame False {
                        n351 = local write "Boolean 4"(FALSE) -> ()
                      }
                      frame True {
                        (unwired) 300
                        n352 = local write "Boolean 4"(TRUE) -> ()
                      }
                    }
                    n353 = Random Number (0-1)() -> (number: 0 to 1=w843:dbl)
                    n354 = Multiply(x=w843, y=300) -> (x*y=w841:dbl)
                  }
                  frame True {
                    n355 = Add(x=w854, y=36) -> (x+y=w855:i32)
                    n356 = local read "v 4"() -> (w850:dbl)
                    n357 = Subtract(x=w852, y=w850) -> (x-y=w851:dbl)
                  }
                }
                n358 = case shown="True" w721 {
                  tunnel: [0 w840] -> w723
                  tunnel: w724 -> [_ w839]
                  tunnel: [w826 w836] -> w725
                  tunnel: w726 -> [_ w837]
                  frame False {
                    n359 = call "reset_velocity.vi"() -> ("Numeric"=w829:dbl)  [unwired: 11 in]
                    n360 = local write "v 5"(w829) -> ()
                    n361 = Greater?(x=w829, y=0) -> (0:w831:bool)
                    n362 = case shown="True" w831 {
                      frame False {
                        (unwired) 0
                        n363 = local write "Boolean 5"(FALSE) -> ()
                      }
                      frame True {
                        n364 = local write "Boolean 5"(TRUE) -> ()
                      }
                    }
                    n365 = Random Number (0-1)() -> (number: 0 to 1=w827:dbl)
                    n366 = Multiply(x=w827, y=300) -> (x*y=w826:dbl)
                  }
                  frame True {
                    n367 = local read "v 5"() -> (w835:dbl)
                    n368 = Add(x=w839, y=36) -> (x+y=w840:i32)
                    n369 = Subtract(x=w837, y=w835) -> (x-y=w836:dbl)
                  }
                }
                n370 = case shown="True" w720 {
                  tunnel: [0 w825] -> w718
                  tunnel: w717 -> [_ w824]
                  tunnel: [w811 w821] -> w716
                  tunnel: w715 -> [_ w822]
                  frame False {
                    n371 = call "reset_velocity.vi"() -> ("Numeric"=w814:dbl)  [unwired: 11 in]
                    n372 = local write "v 6"(w814) -> ()
                    n373 = Greater?(x=w814, y=0) -> (0:w816:bool)
                    n374 = case shown="False" w816 {
                      frame False {
                        n375 = local write "Boolean 6"(FALSE) -> ()
                      }
                      frame True {
                        (unwired) 300
                        n376 = local write "Boolean 6"(TRUE) -> ()
                      }
                    }
                    n377 = Random Number (0-1)() -> (number: 0 to 1=w813:dbl)
                    n378 = Multiply(x=w813, y=300) -> (x*y=w811:dbl)
                  }
                  frame True {
                    n379 = Add(x=w824, y=36) -> (x+y=w825:i32)
                    n380 = local read "v 6"() -> (w820:dbl)
                    n381 = Subtract(x=w822, y=w820) -> (x-y=w821:dbl)
                  }
                }
                n382 = case shown="True" w697 {
                  tunnel: [0 w780] -> w699
                  tunnel: w700 -> [_ w779]
                  tunnel: [w766 w776] -> w701
                  tunnel: w702 -> [_ w777]
                  frame False {
                    n383 = call "reset_velocity.vi"() -> ("Numeric"=w769:dbl)  [unwired: 11 in]
                    n384 = local write "v 9"(w769) -> ()
                    n385 = Greater?(x=w769, y=0) -> (0:w771:bool)
                    n386 = case shown="True" w771 {
                      frame False {
                        (unwired) 0
                        n387 = local write "Boolean 9"(FALSE) -> ()
                      }
                      frame True {
                        n388 = local write "Boolean 9"(TRUE) -> ()
                      }
                    }
                    n389 = Random Number (0-1)() -> (number: 0 to 1=w768:dbl)
                    n390 = Multiply(x=w768, y=300) -> (x*y=w766:dbl)
                  }
                  frame True {
                    n391 = Add(x=w779, y=36) -> (x+y=w780:i32)
                    n392 = local read "v 9"() -> (w775:dbl)
                    n393 = Subtract(x=w777, y=w775) -> (x-y=w776:dbl)
                  }
                }
                n394 = case shown="False" w750 {
                  tunnel: [0 w900] -> w748
                  tunnel: w747 -> [_ w899]
                  tunnel: [w886 w896] -> w746
                  tunnel: w745 -> [_ w897]
                  frame False {
                    # "reser velocity"
                    n395 = call "reset_velocity.vi"() -> ("Numeric"=w889:dbl)  [unwired: 11 in]
                    n396 = local write "v"(w889) -> ()
                    n397 = Greater?(x=w889, y=0) -> (0:w891:bool)
                    n398 = case shown="False" w891 {
                      frame False {
                        n399 = local write "Boolean"(FALSE) -> ()
                      }
                      frame True {
                        n400 = local write "Boolean"(TRUE) -> ()
                      }
                    }
                    n401 = Random Number (0-1)() -> (number: 0 to 1=w888:dbl)
                    n402 = Multiply(x=w888, y=300) -> (x*y=w886:dbl)
                  }
                  frame True {
                    n403 = Add(x=w899, y=36) -> (x+y=w900:i32)
                    n404 = local read "v"() -> (w895:dbl)
                    n405 = Subtract(x=w897, y=w895) -> (x-y=w896:dbl)
                  }
                }
                n406 = call "tree_move.vi"("Left in"=w675, "Top"=w676) -> ("Numeric"=w667:i32, "Left out"=w668:dbl)  [unwired: 8 in]
                n407 = call "tree_move.vi"("Left in"=w680, "Top"=w679) -> ("Numeric"=w671:i32, "Left out"=w672:dbl)  [unwired: 8 in]
                n408 = call "tree_move.vi"("Left in"=w677, "Top"=w678) -> ("Numeric"=w669:i32, "Left out"=w670:dbl)  [unwired: 8 in]
                n409 = call "tree_move.vi"("Left in"=w682, "Top"=w681) -> ("Numeric"=w673:i32, "Left out"=w674:dbl)  [unwired: 8 in]
                n410 = call "tree_move.vi"("Left in"=w685, "Top"=w686) -> ("Numeric"=w684:i32, "Left out"=w683:dbl)  [unwired: 8 in]
                n411 = Increment(x=w688) -> (x+1=w687:i16)
                n412 = property on="Boolean 11" class="Bool (strict)"("Visible"=TRUE) -> ()  [unwired: 2 in, 2 out]
              }
            }
          }
        }
        n413 = property on="tree 5" class="Bool"("Left"=w193, "Top"=w202) -> ()  [unwired: 2 in, 2 out]
        n414 = property on="tree 3" class="Bool"("Left"=w195, "Top"=w204) -> ()  [unwired: 2 in, 2 out]
        n415 = property on="tree 4" class="Bool"("Left"=w194, "Top"=w203) -> ()  [unwired: 2 in, 2 out]
        n416 = property on="tree" class="Bool"("Left"=w197, "Top"=w214) -> ()  [unwired: 2 in, 2 out]
        n417 = property on="tree 2" class="Bool"("Left"=w196, "Top"=w205) -> ()  [unwired: 2 in, 2 out]
        n418 = property on="chicken" class="Bool"("Left"=w220) -> ()  [unwired: 2 in, 2 out]
        n419 = property on="Boolean 2" class="Bool (strict)"("Left"=w245, "Top"=w273) -> ()  [unwired: 2 in, 2 out]
        n420 = property on="Boolean 4" class="Bool (strict)"("Left"=w243, "Top"=w266) -> ()  [unwired: 2 in, 2 out]
        n421 = property on="Boolean 5" class="Bool (strict)"("Left"=w242, "Top"=w264) -> ()  [unwired: 2 in, 2 out]
        n422 = property on="Boolean 3" class="Bool (strict)"("Left"=w244, "Top"=w269) -> ()  [unwired: 2 in, 2 out]
        n423 = property on="Boolean 6" class="Bool (strict)"("Left"=w241, "Top"=w261) -> ()  [unwired: 2 in, 2 out]
        n424 = property on="Boolean 8" class="Bool (strict)"("Left"=w239, "Top"=w254) -> ()  [unwired: 2 in, 2 out]
        n425 = property on="Boolean 7" class="Bool (strict)"("Left"=w240, "Top"=w259) -> ()  [unwired: 2 in, 2 out]
        n426 = property on="Boolean 9" class="Bool (strict)"("Left"=w238, "Top"=w251) -> ()  [unwired: 2 in, 2 out]
        n427 = property on="Boolean 10" class="Bool (strict)"("Left"=w237, "Top"=w248) -> ()  [unwired: 2 in, 2 out]
        n428 = property on="Boolean" class="Bool (strict)"("Left"=w246, "Top"=w272) -> ()  [unwired: 2 in, 2 out]
        n429 = Quotient & Remainder(x=w201, y=w199) -> (x-y*floor(x/y)=w200:i16)  [unwired: 1 out]
        n430 = Subtract(x=w199, y=w200) -> (x-y=w198:i16)
        n431 = case shown="2, 4, 6, 8, 10, Default" w198 {
          tunnel: [10000 w280 w281 w282 w283 w284] -> w191
          tunnel: w197 -> [_ w280 _ _ _ _]
          tunnel: w196 -> [_ _ w281 _ _ _]
          tunnel: w195 -> [_ _ _ w282 _ _]
          tunnel: w194 -> [_ _ _ _ w283 _]
          tunnel: w193 -> [_ _ _ _ _ w284]
          frame 2, 4, 6, 8, 10, Default {
          }
          frame 1 {
          }
          frame 3 {
          }
          frame 5 {
          }
          frame 7 {
          }
          frame 9 {
          }
        }
        n432 = Quotient & Remainder(x=w201, y=i16 10) -> (x-y*floor(x/y)=w234:i16)  [unwired: 1 out]
        n433 = Subtract(x=i16 10, y=w234) -> (x-y=w228:i16)
        n434 = property on="chicken" class="Bool"() -> ("Left"=w192:i32)  [unwired: 2 in, 2 out]
        n435 = case shown="1" w228 {
          tunnel: w246 -> [_ w303 _ _ _ _ _ _ _ _]
          tunnel: w245 -> [_ _ w304 _ _ _ _ _ _ _]
          tunnel: w244 -> [_ _ _ w305 _ _ _ _ _ _]
          tunnel: w243 -> [_ _ _ _ w306 _ _ _ _ _]
          tunnel: w242 -> [_ _ _ _ _ w307 _ _ _ _]
          tunnel: w241 -> [_ _ _ _ _ _ w308 _ _ _]
          tunnel: w240 -> [_ _ _ _ _ _ _ w309 _ _]
          tunnel: w239 -> [_ _ _ _ _ _ _ _ w310 _]
          tunnel: w238 -> [_ _ _ _ _ _ _ _ _ w311]
          tunnel: w237 -> [w302 _ _ _ _ _ _ _ _ _]
          tunnel: [w302 w303 w304 w305 w306 w307 w308 w309 w310 w311] -> w224
          frame 10, Default {
          }
          frame 1 {
          }
          frame 2 {
          }
          frame 3 {
          }
          frame 4 {
          }
          frame 5 {
          }
          frame 6 {
          }
          frame 7 {
          }
          frame 8 {
          }
          frame 9 {
          }
        }
        n436 = local write "SCORE"(w201) -> ()
        n437 = Subtract(x=w192, y=w191) -> (x-y=w190:dbl)
        n438 = local read "easy?"() -> (w186:bool)
        n439 = In Range and Coerce(upper limit=24.0, x=w190, lower limit=-24.0) -> (In Range?=w187:bool)  [unwired: 1 out]
        n440 = property on="chicken" class="Bool"() -> ("Left"=w232:i32)  [unwired: 2 in, 2 out]
        n441 = And(x=w187, y=w186) -> (x .and. y?=w183:bool)
        n442 = Quotient & Remainder(x=w228, y=i16 2) -> (x-y*floor(x/y)=w226:i16)  [unwired: 1 out]
        n443 = local read "easy?"() -> (w219:bool)
        n444 = Greater Than 0?(x=w226) -> (x > 0?=w225:bool)
        n445 = And(x=w219, y=w225) -> (x .and. y?=w218:bool)
        n446 = Select(t=10000.0, s=w218, f=w224) -> (s? t:f=w222:dbl)
        n447 = Subtract(x=w232, y=w222) -> (x-y=w231:dbl)
        n448 = In Range and Coerce(upper limit=i16 54 ("lower limit"), x=w231, lower limit=i16 -24) -> (In Range?=w185:bool)  [unwired: 1 out]
        n449 = Or(x=w185, y=w183) -> (x .or. y?=w184:bool)
        n450 = case shown="True" w184 {
          tunnel: w201 -> [_ w299]
          tunnel: [FALSE TRUE] -> w235
          frame False {
          }
          frame True {
            # "game over"
            # "reset top score"
            n451 = local read "TOP"() -> (w300:i16)
            n452 = property on="Boolean 12" class="Bool (strict)"("Visible"=TRUE) -> ()  [unwired: 2 in, 2 out]
            n453 = Greater?(x=w299, y=w300) -> (0:w301:bool)
            n454 = Select(t=w299, s=w301, f=w300) -> (s? t:f=w298:i16)
            n455 = local write "TOP"(w298) -> ()
          }
        }
        n456 = case shown="False" w218 {
          frame False {
            # "move the grass"
            n457 = property on="grass 1" class="Bool"("Top"=0) -> ()  [unwired: 2 in, 2 out]
            n458 = property on="grass 2" class="Bool"("Top"=72) -> ()  [unwired: 2 in, 2 out]
            n459 = property on="grass 3" class="Bool"("Top"=144) -> ()  [unwired: 2 in, 2 out]
            n460 = property on="grass 4" class="Bool"("Top"=216) -> ()  [unwired: 2 in, 2 out]
            n461 = property on="grass 5" class="Bool"("Top"=288) -> ()  [unwired: 2 in, 2 out]
          }
          frame True {
            n462 = property on="grass 1" class="Bool"("Top"=36) -> ()  [unwired: 2 in, 2 out]
            n463 = property on="grass 2" class="Bool"("Top"=108) -> ()  [unwired: 2 in, 2 out]
            n464 = property on="grass 3" class="Bool"("Top"=180) -> ()  [unwired: 2 in, 2 out]
            n465 = property on="grass 4" class="Bool"("Top"=252) -> ()  [unwired: 2 in, 2 out]
            n466 = property on="grass 5" class="Bool"("Top"=324) -> ()  [unwired: 2 in, 2 out]
          }
        }
        n467 = call <vilib>:"Sound Output Info.vi"("task ID"=w181) -> ("task ID out"=w180:T8)  [unwired: 7 in, 3 out]
        n468 = Or(x=w235, y="stop") -> (x .or. y?=w182:bool)
      }
      n469 = property on="v" class="DigNum (strict)"("Visible"=w98) -> ()  [unwired: 2 in, 2 out]
      n470 = property on="v 2" class="DigNum (strict)"("Visible"=w98) -> ()  [unwired: 2 in, 2 out]
      n471 = property on="v 3" class="DigNum (strict)"("Visible"=w98) -> ()  [unwired: 2 in, 2 out]
      n472 = property on="v 4" class="DigNum (strict)"("Visible"=w98) -> ()  [unwired: 2 in, 2 out]
      n473 = property on="v 5" class="DigNum (strict)"("Visible"=w98) -> ()  [unwired: 2 in, 2 out]
      n474 = property on="v 6" class="DigNum (strict)"("Visible"=w98) -> ()  [unwired: 2 in, 2 out]
      n475 = property on="v 7" class="DigNum (strict)"("Visible"=w98) -> ()  [unwired: 2 in, 2 out]
      n476 = property on="v 8" class="DigNum (strict)"("Visible"=w98) -> ()  [unwired: 2 in, 2 out]
      n477 = property on="v 9" class="DigNum (strict)"("Visible"=w98) -> ()  [unwired: 2 in, 2 out]
      n478 = property on="v 10" class="DigNum (strict)"("Visible"=w98) -> ()  [unwired: 2 in, 2 out]
      n479 = local write "SCORE"(i16 0 ("score")) -> ()
      n480 = call <vilib>:"Sound Output Clear.vi"("task ID"=w60) -> ()  [unwired: 10 in, 1 out]
    }
  }
  n481 = property on="EASY" class="Bool"("Visible"=w8) -> ()  [unwired: 2 in, 2 out]
  n482 = property on="HARD" class="Bool"("Visible"=w8) -> ()  [unwired: 2 in, 2 out]
  n483 = property on="Boolean 12" class="Bool (strict)"("Visible"=FALSE, "Value"=T1 FALSE ("Boolean 12")) -> ()  [unwired: 2 in, 2 out]
  n484 = property on="Boolean 11" class="Bool (strict)"("Visible"=FALSE) -> ()  [unwired: 2 in, 2 out]
